vi "CLK.vi"(0 "Frequency":dbl) -> (1 "CLK":bool, 2 "_____\nCLK":bool)   [LabVIEW 2018]
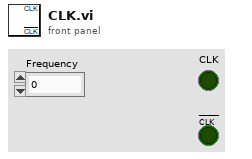
[diagram p1: front panel]
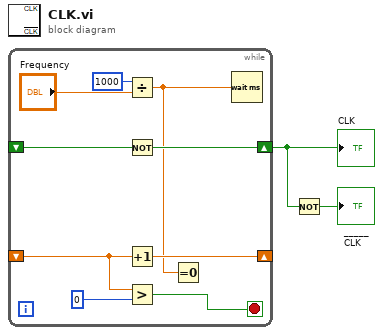
[diagram p0: block diagram]
diagram:
  n1 = while {
    shift-right: [w8] -> w1
    shift-left: _ -> [w9]
    shift-right: [w7] -> _
    shift-left: _ -> [w6]
    stop <- w5 stop-if-true
    n2 = Divide(x=1000, y="Frequency") -> (x/y=w3:dbl)
    n3 = Not(x=w9) -> (.not. x?=w8:bool)
    n4 = Increment(x=w6) -> (x+1=w7:dbl)
    n5 = Greater?(x=w6, y=0) -> (0:w5:bool)
    n6 = Equal To 0?(x=w3) -> ()  [unwired: 1 out]
    n7 = Wait (ms)(milliseconds to wait=w3) -> ()  [unwired: 1 out]
  }
  "CLK" <- w1
  n8 = Not(x=w1) -> (.not. x?=→"_____\nCLK":bool)
